vi "firma.vi"() -> ()   [LabVIEW 2016]
uses:
  <vilib>/Utility/miscctls.llb/LVMouseTypeDef.ctl
panel:
  out "XY Graph":cluster{i32[], i32[]}(graph)
  out "Waveform Graph 2":i32[](graph)
  out "Waveform Graph":i32[](graph)
  out "Mouse":T1
  in  "Stop Button":bool
  in  "pen":T2={"Width"=1, "Style"=enum."Solid"}
  out "new picture":picture
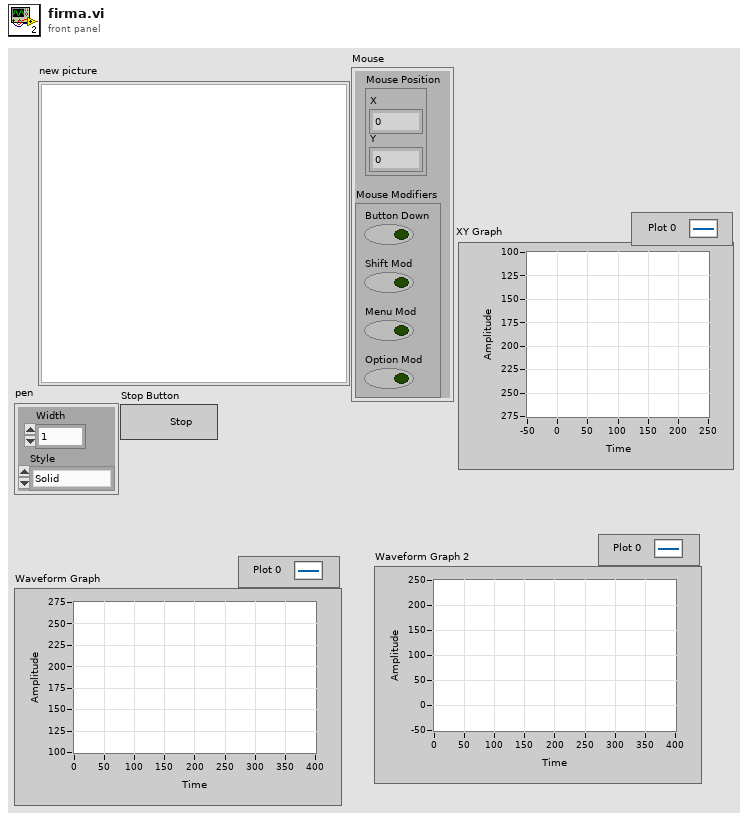
[diagram p1: front panel]
types:
  T1 = typedef "LVMouseTypeDef.ctl" = cluster{"Mouse Position":cluster{"X":i32, "Y":i32}, "Mouse Modifiers":cluster{"Button Down":bool, "Shift Mod":bool, "Menu Mod":bool, "Option Mod":bool}}
  T2 = cluster{"Width":u16, "Style":enum32{"Solid", "Dash", "Dot", "DashDot", "DashDotDot"}}
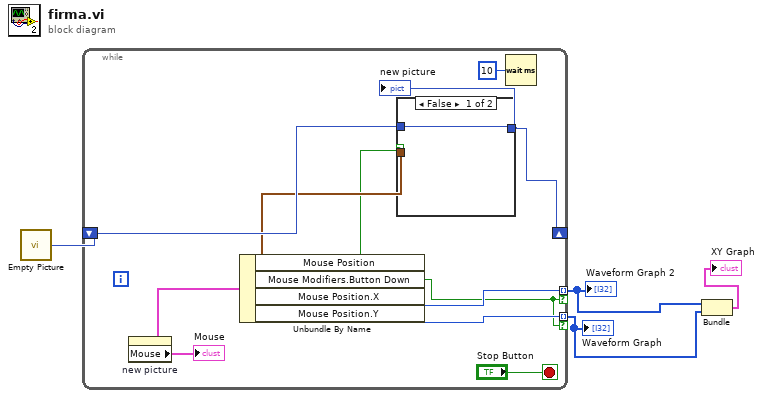
[diagram p0: block diagram]
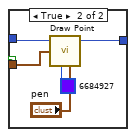
[diagram p2: hidden frame]
diagram:
  n1 = call "Empty Picture"() -> ("empty picture"=w4:picture)
  n2 = while {
    shift-right: [w11] -> _
    shift-left: w4 -> [w10]
    tunnel: [w7] -> w3 mode=indexing if=w5
    tunnel: [w6] -> w2 mode=indexing if=w5
    stop <- "Stop Button" stop-if-true
    n3 = property on="new picture" class="Pict"() -> ("Mouse"=w9:T1)  [unwired: 2 in, 2 out]
    "Mouse" <- w9
    n4 = Unbundle By Name(w9) -> ("Mouse Position"=w8:cluster{"X":i32, "Y":i32}, "Mouse Modifiers.Button Down"=w5:bool, "Mouse Position.X"=w7:i32, "Mouse Position.Y"=w6:i32)
    n5 = case shown="False" w5 {
      tunnel: [w14 w17] -> w11
      tunnel: w10 -> [w14 w16]
      tunnel: w8 -> [_ w15]
      frame False {
      }
      frame True {
        n6 = call <vilib>:"Draw Point.vi"("picture"=w16, "point(x,y)"=w15, "color(black)"=u32 6684927, "pen"="pen") -> ("new picture"=w17:picture)  [unwired: 5 in]
      }
    }
    "new picture" <- w11
    n7 = Wait (ms)(milliseconds to wait=u32 10) -> ()  [unwired: 1 out]
  }
  "Waveform Graph" <- w2
  "Waveform Graph 2" <- w3
  n8 = Bundle(w3, w2) -> (→"XY Graph":cluster{i32[], i32[]})  [unwired: 1 in]
